vi "Get Thermocouple Meas Value.vi"(8 "error in (no error)":errorcluster, 11 "VISA resource name":refnum<visa-resource-name>) -> (0 "error out":errorcluster {"code" format="%.0x"}, 1 "Value Units":i32, 2 "Meas Value":dbl format="%^.3e", 3 "VISA resource name out":refnum<visa-resource-name>)   [LabVIEW 2011, in "Fluke 5XXX Series Multicalibrators.lvlib"]
doc: "This VI returns the last value of the thermocouple measurement. The unit returns indicates the status of the reading. Returns 0 and NONE when there is no recent measurement either because the Calibrator is not in a measurement mode, or because no measurement has been made yet.\n\nNote:\n\nThis VI is available only for instrument models 5500A and 5520A."
uses:
  Fluke 5XXX Series Multicalibrators.lvlib
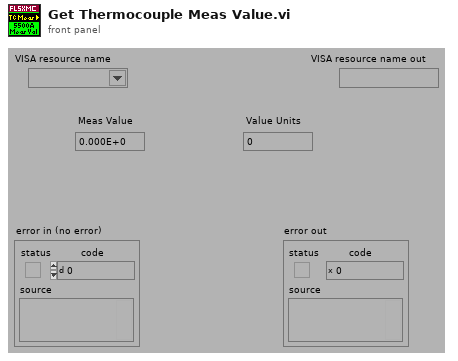
[diagram p1: front panel]
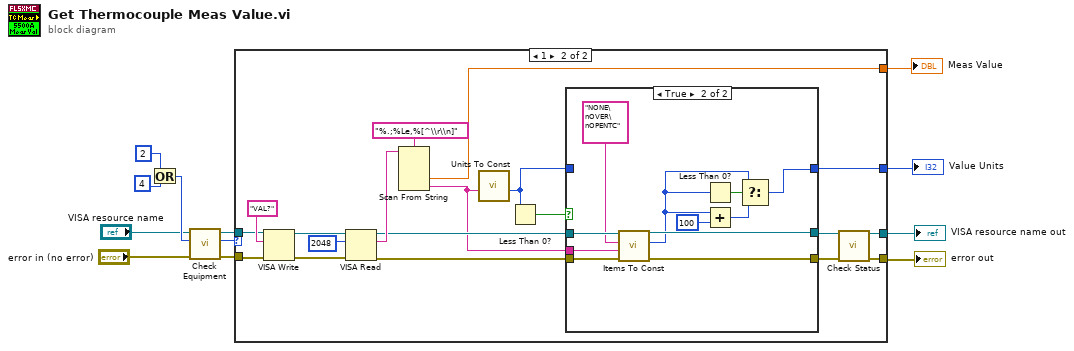
[diagram p0: block diagram]
diagram:
  n1 = Or(x=2 ("Numeric"), y=4 ("Numeric")) -> (x .or. y?=w8:i32)
  n2 = call "Check Equipment.vi"("error in (no error)"="error in (no error)", "Bit Mask"=w8, "VISA resource name"="VISA resource name") -> ("error out"=w12:errorcluster, "Present?"=w11:u32, "VISA resource name out"=w1:refnum<visa-resource-name>)  [unwired: 6 in]
  n3 = case shown="1" w11 {
    tunnel: [w16 w30] -> w5
    tunnel: [w13 w29] -> w4
    tunnel: w12 -> [w16 w31]
    tunnel: [0.0 w26] -> w3
    tunnel: [0 w24] -> w7
    tunnel: w1 -> [w13 w18]
    frame 0, Default {
    }
    frame 1 {
      n4 = VISA Write(VISA resource name=w18, write buffer="VAL?", error in (no error)=w31) -> (VISA resource name out=w34:refnum<visa-resource-name>, error out=w33:errorcluster)  [unwired: 1 out]
      n5 = VISA Read(VISA resource name=w34, byte count=u32 2048 ("byte count (0)"), error in (no error)=w33) -> (VISA resource name out=w23:refnum<visa-resource-name>, read buffer=w27:string, error out=w20:errorcluster)  [unwired: 1 out]
      n6 = Scan From String(format string="%.;%Le,%[^\\r\\n]", input string=w27) -> (output 1=w26:dbl, output 2=w19:string)  [unwired: 4 in, 3 out]
      n7 = call "Units To Const.vi"("Units"=w19) -> ("Const"=w17:i32)  [unwired: 10 in]
      n8 = Less Than 0?(x=w17) -> (x < 0?=w25:bool)
      n9 = case shown="True" w25 {
        tunnel: w17 -> [w38 _]
        tunnel: [w38 w45] -> w24
        tunnel: w23 -> [w36 w48]
        tunnel: [w36 w49] -> w22
        tunnel: [w37 w40] -> w21
        tunnel: w20 -> [w37 w42]
        tunnel: w19 -> [_ w46]
        frame False {
        }
        frame True {
          n10 = call "Items To Const.vi"("error in (no error)"=w42, "String Item"=w46, "Multi-Line String"="NONE\nOVER\nOPENTC", "VISA resource name"=w48) -> ("error out"=w40:errorcluster, "Index"=w39:i32, "VISA resource name out"=w49:refnum<visa-resource-name>)  [unwired: 5 in]
          n11 = Less Than 0?(x=w39) -> (x < 0?=w41:bool)
          n12 = Add(x=w39, y=100) -> (x+y=w44:i32)
          n13 = Select(t=w39, s=w41, f=w44) -> (s? t:f=w45:i32)
        }
      }
      n14 = call "Check Status.vi"("VISA resource name"=w22, "error in (no error)"=w21) -> ("VISA resource name out"=w29:refnum<visa-resource-name>, "error out"=w30:errorcluster)  [unwired: 12 in]
    }
  }
  "Meas Value" <- w3
  "Value Units" <- w7
  "VISA resource name out" <- w4
  "error out" <- w5
